vi "AMI.vi"(1 "输入":i8[](array[numeric])) -> (0 "输出":i8[](array[numeric]))   [LabVIEW 2018]
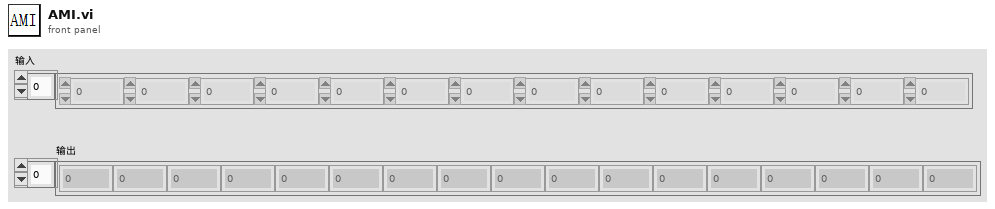
[diagram p1: front panel]
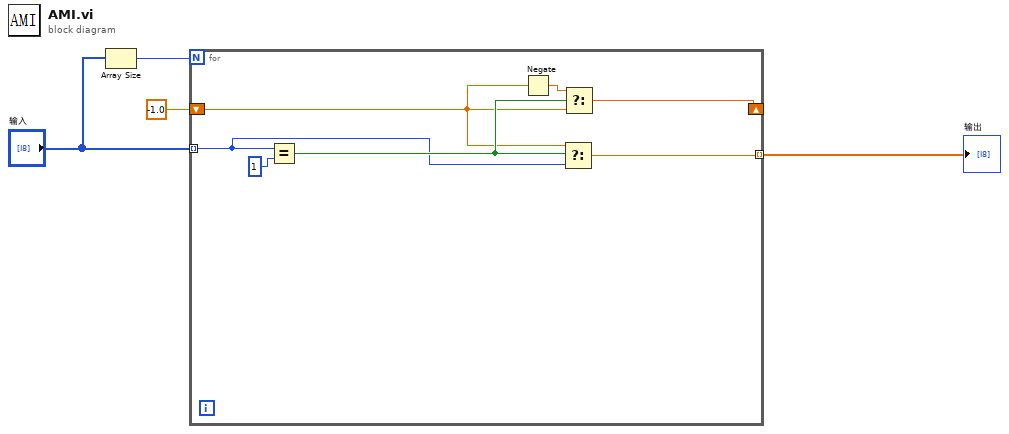
[diagram p0: block diagram]
diagram:
  n1 = Array Size(array="输入") -> (size(s)=w3:i32)
  n2 = for {
    N: w3 -> [_]
    tunnel: "输入" -> [w5] mode=indexing
    shift-right: [w8] -> _
    shift-left: -1.0 -> [w6]
    tunnel: [w9] -> w1 mode=indexing
    n3 = Equal?(x=w5, y=i8 1) -> (x = y?=w10:bool)
    n4 = Negate(x=w6) -> (-x=w7:dbl)
    n5 = Select(t=w6, s=w10, f=w5) -> (s? t:f=w9:dbl)
    n6 = Select(t=w7, s=w10, f=w6) -> (s? t:f=w8:dbl)
  }
  "输出" <- w1
